vi "Creat insert cmd.vi"(7 "Data":string[](array[string]), 8 "error in (no error)":errorcluster, 9 "columns":string[](array[string]), 10 "num parameters":i32, 11 "table name":string) -> (0 "error out":errorcluster, 3 "insert query":string)   [LabVIEW 2014]
uses:
  <vilib>/addons/database/NI_Database_API.lvlib
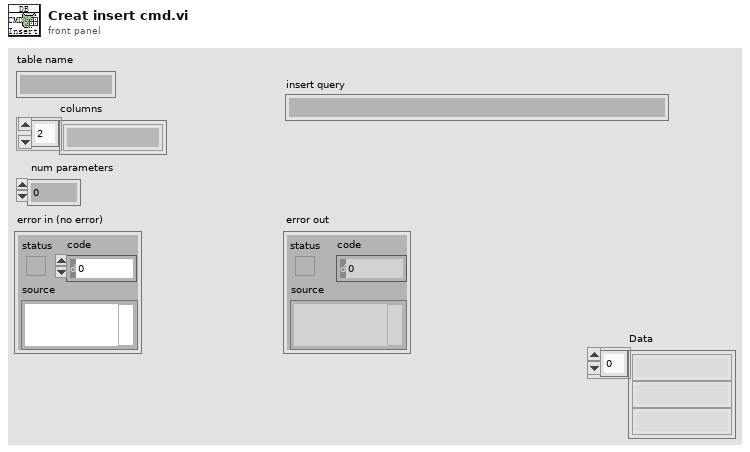
[diagram p1: front panel]
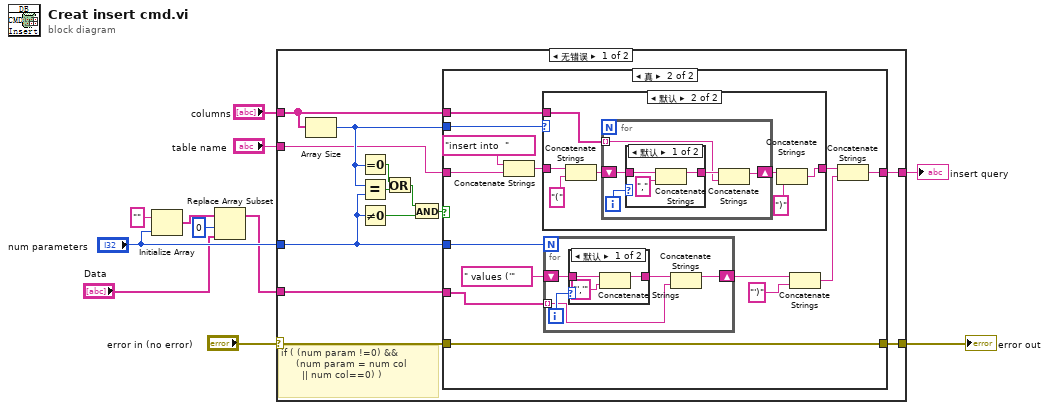
[diagram p0: block diagram]
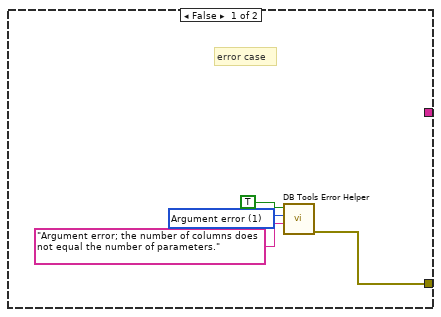
[diagram p2: hidden frame]
diagram:
  n1 = Initialize Array("", "num parameters") -> (w4:string[])
  n2 = Replace Array Subset(array=w4, new element="Data", index=0 ("索引")) -> (w1:string[])
  n3 = case shown="无错误" "error in (no error)" {
    selector: "error in (no error)" -> [w18 w69]
    tunnel: [w17 w69] -> w10
    tunnel: "columns" -> [w16 _]
    tunnel: "num parameters" -> [w15 _]
    tunnel: [w14 _] -> w8
    tunnel: "table name" -> [w13 _]
    tunnel: w1 -> [w12 _]
    frame No Error {
      # "if ( (num param !=0) &&\n     (num param = num col \n       || num col==0) )"
      n4 = Array Size(array=w16) -> (size(s)=w19:i32)
      n5 = Equal To 0?(x=w19) -> (x = 0?=w24:bool)
      n6 = Equal?(x=w19, y=w15) -> (x = y?=w20:bool)
      n7 = Not Equal To 0?(x=w15) -> (x != 0?=w23:bool)
      n8 = Or(x=w24, y=w20) -> (x .or. y?=w22:bool)
      n9 = And(x=w22, y=w23) -> (x .and. y?=w21:bool)
      n10 = case shown="真" w21 {
        tunnel: w16 -> [_ w39]
        tunnel: w19 -> [_ w38]
        tunnel: w15 -> [_ w36]
        tunnel: w18 -> [_ w32]
        tunnel: [w28 w32] -> w17
        tunnel: [_ w31] -> w14
        tunnel: w13 -> [_ w30]
        tunnel: w12 -> [_ w29]
        frame False {
          w26 = 1 items=["No error", "Argument error", "Memory is full", "Out of zone", "End of file", "File already open", "Generic file I/O error", "File not found", "File permission error", "Disk is full", "Duplicate path", "Too many files open", "System feature not enabled", "Resource file not found", "Cannot add resource", "Resource not found", "Image not found", "Image memory error", "Pen does not exist", "Config type invalid", "Config token not found", "Config parse error", "Config memory error", "Bad external code format", "Bad external code offset", "External code not present", "Null window", "Destroy window error", "Null menu", "Print aborted", "Bad print record", "Print driver error", "Windows error during printing", "Memory error during printing", "Print dialog error", "Generic print error", "Invalid device refnum", "Device not found", "Device parameter error", "Device unit error", "Cannot open device", "Device call aborted", "Generic error", "Cancelled by user", "Object ID too low", "Object ID too high", "Object not in heap", "Unknown heap", "Unknown object (invalid DefProc)", "Unknown object (DefProc not in table)", "Message out of range", "Invalid (null) method", "Unknown message", "Manager call not supported", "Bad address", "Network operation in progress", "Network operation timed out", "Connection is busy", "Network attribute not supported", "Network error", "Address in use", "System out of memory", "Connection aborted", "Connection refused", "Not connected", "Already connected", "Connection closed", "Initialization error (interapplication manager)", "Bad occurrence", "Wait on unbound occurrence handler", "Occurrence queue overflow", "Datalog type conflict", "Unused", "Unrecognized type (interapplication manager)", "Memory corrupt", "Failed to make temporary DLL", "Old CIN version", "Drag socket not found", "Failed to load drop-object", "Failed to register OLE object", "Failed to release OLE object", "Format specifier type mismatch", "Unknown format specifier", "Too few format specifiers", "Too many format specifiers", "Scan failed", "Newer CIN version", "Error converting to variant", "Runtime menu error", "Password tampered", "Variant attribute not found", "Incompatible variant data type", "Event data is not available", "Event Store is not present", "Occurrence is not found", "Event Queue is not created", "Event info is not available", "Refnum passed is NULL", "Error retrieving Class GUID", "Error retrieving CoClass GUID", "Error retrieving TypeLib GUID.", "Bad built application magic bytes.", "Specific driver is different from the specific driver associated with the Logical Name.", "There is no session opened to the class driver.", "Max Error", "MAX - Error with config objects", "MAX - Error loading configuration", "MAX - Group not supported"]
          # "error case"
          n11 = call <vilib>:"DB Tools Error Helper.vi"("source"="Argument error; the number of columns does not equal the number of parameters.", "code"=w26, "status"=TRUE) -> ("error out"=w28:errorcluster)  [unwired: 1 in, 7 out]
        }
        frame True {
          n12 = Concatenate Strings("insert into  " ("Substring"), w30) -> (w41:string)
          n13 = case shown="默认" w38 {
            tunnel: w39 -> [_ w59]
            tunnel: [w52 w53] -> w42
            tunnel: w41 -> [w52 w58]
            frame 0 {
              # "if the columns\narray is empty"
            }
            frame Default {
              n14 = Concatenate Strings(w58, "(" ("Substring")) -> (w56:string)
              n15 = for {
                tunnel: w59 -> [w61] mode=indexing
                shift-right: [w60] -> w55
                shift-left: w56 -> [w63]
                i -> [w64]
                n16 = case shown="默认" w64 {
                  tunnel: w63 -> [w67 w68]
                  tunnel: [w65 w68] -> w62
                  frame Default {
                    n17 = Concatenate Strings(w67, "," ("Substring")) -> (w65:string)
                  }
                  frame 0 {
                  }
                }
                n18 = Concatenate Strings(w62, w61) -> (w60:string)
              }
              n19 = Concatenate Strings(w55, ")" ("Substring")) -> (w53:string)
            }
          }
          n20 = for {
            N: w36 -> [_]
            shift-right: [w44] -> w34
            shift-left: " values ('" ("Substring") -> [w46]
            tunnel: w29 -> [w43] mode=indexing
            i -> [w47]
            n21 = case shown="默认" w47 {
              tunnel: w46 -> [w50 w51]
              tunnel: [w48 w51] -> w45
              frame Default {
                n22 = Concatenate Strings(w50, "','" ("Substring")) -> (w48:string)
              }
              frame 0 {
              }
            }
            n23 = Concatenate Strings(w45, w43) -> (w44:string)
          }
          n24 = Concatenate Strings(w34, "')" ("Substring")) -> (w33:string)
          n25 = Concatenate Strings(w42, w33) -> (w31:string)
        }
      }
    }
    frame Error {
    }
  }
  "error out" <- w10
  "insert query" <- w8
